vi "IQ Impairments.vi"(0 "data in":T1[](array[typedef])=[{"I"=0.0, "Q"=0.0, "overflow"=FALSE}, {"I"=0.0, "Q"=0.0, "overflow"=FALSE}], 9 "input valid":bool, 11 "acq in":refnum<class "niUSRP Rx DSP v2 FPGA.lvclass">, 12 "ready for output (T)":bool=TRUE) -> (4 "data out":T1[](array[typedef]), 10 "output valid":bool, 14 "ready for input":bool, 15 "acq out":refnum<class "niUSRP Rx DSP v2 FPGA.lvclass">)   [LabVIEW 2025, in "niUSRP Rx DSP v2 FPGA.lvclass"]
uses:
  niUSRP Rx DSP v2 FPGA.lvclass
  <instrlib>/_niInstr/DSP/v1/Shared/Public/IQ Data.ctl
  <instrlib>/_niInstr/DSP Control/Interface/v1/FPGA/IQ Impairments/IQ 18-bit/IQ Impairments Interface (18-bit).lvclass
  <instrlib>/_niInstr/Basic Elements/v1/FPGA/niInstr Basic Elements v1 FPGA.lvlib
  <instrlib>/_niInstr/DSP/v1/Shared/niInstr DSP v1 Shared.lvlib
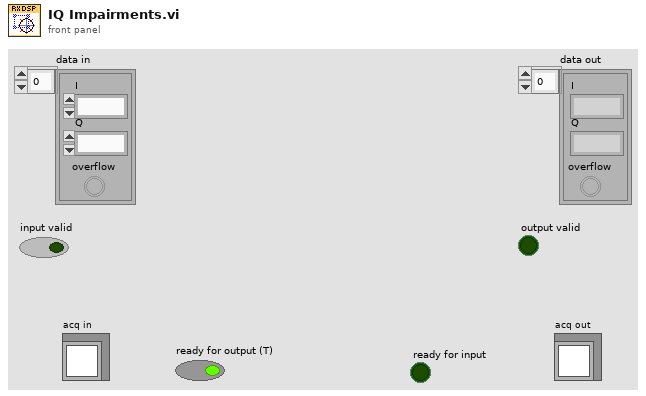
[diagram p1: front panel]
types:
  T1 = typedef "niInstr DSP v1 Shared.lvlib/IQ Data.ctl" = cluster{"I":fxp<+/-,18,1>, "Q":fxp<+/-,18,1>, "overflow":bool}
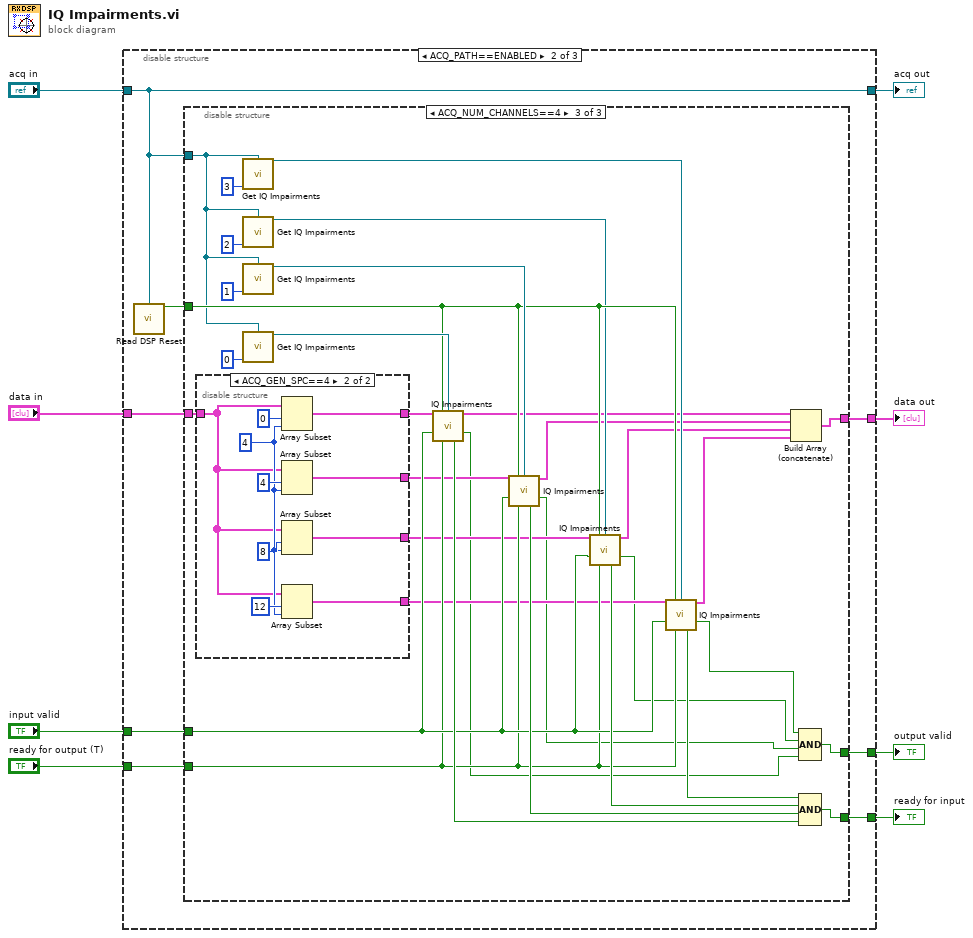
[diagram p0: block diagram]
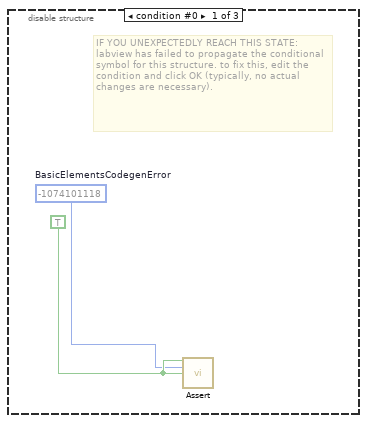
[diagram p2: hidden frame]
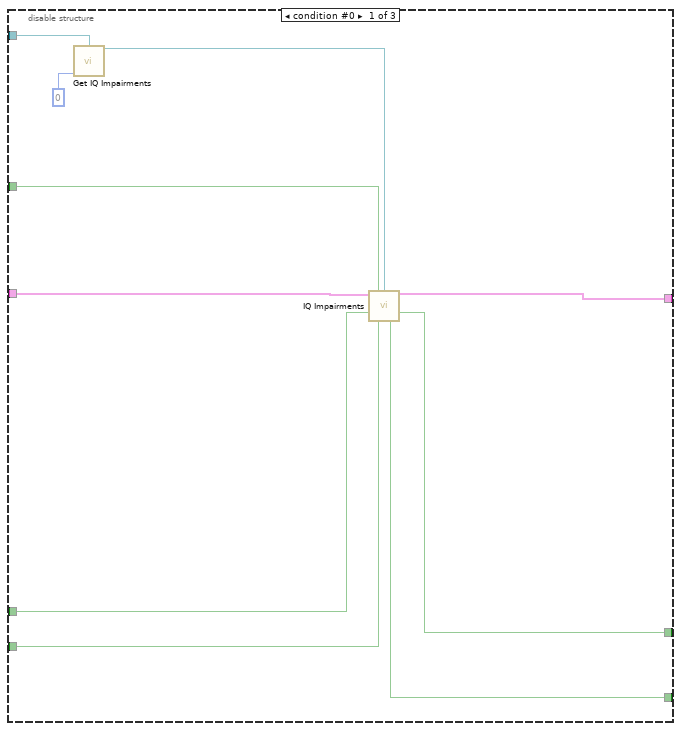
[diagram p3: hidden frame]
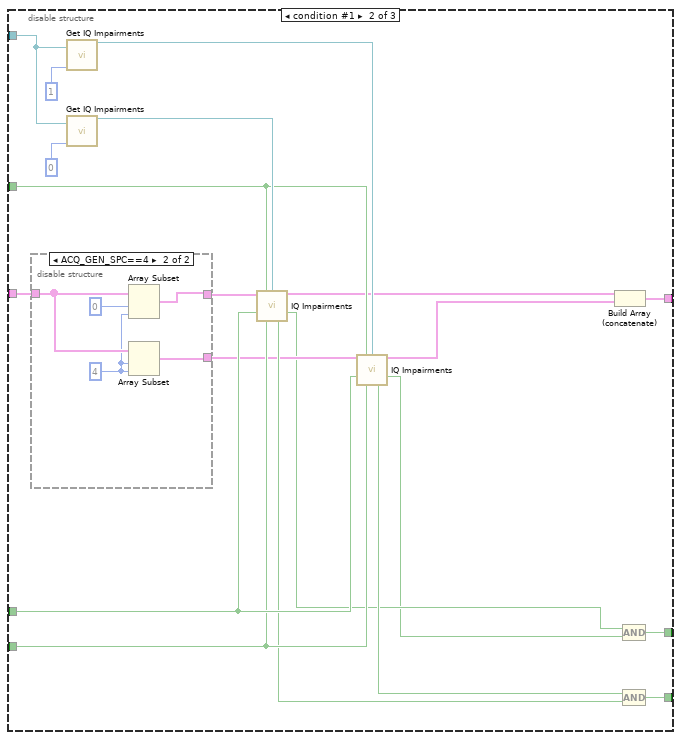
[diagram p4: hidden frame]
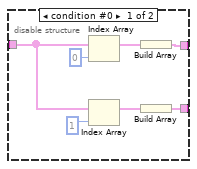
[diagram p5: hidden frame]
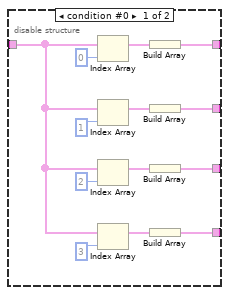
[diagram p6: hidden frame]
diagram:
  n1 = disable-structure shown="ACQ_PATH==ENABLED" {
    disable-tunnel: [_ w18 w118] -> w8
    disable-tunnel: "input valid" -> [_ w17 w116]
    disable-tunnel: "ready for output (T)" -> [_ w16 w117]
    disable-tunnel: [_ w15 w116] -> w5
    disable-tunnel: "acq in" -> [_ w12 w119]
    disable-tunnel: [_ w12 w119] -> w4
    disable-tunnel: "data in" -> [_ w11 w118]
    disable-tunnel: [_ w14 w117] -> w2
    frame condition #0 {
      w10 = TRUE ("assert")
      w9 = -1074101118  # BasicElementsCodegenError
      # "IF YOU UNEXPECTEDLY REACH THIS STATE:\nlabview has failed to propagate the conditional symbol for this structure. to fix this, edit the condition and click OK (typically, no actual changes are necessary)."
      n2 = call <instrlib>:"Assert.vi"("assert"=w10, "error code"=w9, "enable show error"=w10) -> ()  [unwired: 13 in]
    }
    frame condition #1 (active) {
      n3 = call-dynamic "Read DSP Reset.vi"("acq"=w12) -> ("dsp reset"=w13:bool)  [unwired: 14 in]
      n4 = disable-structure shown="ACQ_NUM_CHANNELS==4" {
        disable-tunnel: [w28 w40 w88] -> w18
        disable-tunnel: w17 -> [w27 w42 w76]
        disable-tunnel: w16 -> [w26 w41 w75]
        disable-tunnel: [w25 w39 w87] -> w15
        disable-tunnel: [w24 w38 w86] -> w14
        disable-tunnel: w13 -> [w23 w43 w81]
        disable-tunnel: w12 -> [w21 w45 w74]
        disable-tunnel: w11 -> [w19 w35 w73]
        frame condition #0 {
          n5 = call-dynamic "Get IQ Impairments.vi"("acq in"=w21, "ch"=u8 0) -> ("iq impairments"=w22:refnum<class "IQ Impairments Interface (18-bit).lvclass">)  [unwired: 13 in]
          n6 = call-dynamic "IQ Impairments.vi"("data in"=w19, "reset"=w23, "iq impairments"=w22, "input valid"=w27, "ready for output (T)"=w26) -> ("data out"=w28:T1[], "output valid"=w25:bool, "ready for input"=w24:bool)  [unwired: 7 in, 1 out]
        }
        frame condition #1 {
          n7 = disable-structure shown="ACQ_GEN_SPC==4" {
            disable-tunnel: w35 -> [w51 w58]
            disable-tunnel: [w50 w59] -> w34
            disable-tunnel: [w49 w57] -> w33
            frame condition #0 {
              n8 = Index Array(array=w51, index=0) -> (element=w55:T1)
              n9 = Index Array(array=w51, index=1) -> (element=w53:T1)
              n10 = Build Array(w55) -> (w50:T1[])
              n11 = Build Array(w53) -> (w49:T1[])
            }
            frame condition #1 (active) {
              w56 = 4 ("length")
              n12 = Array Subset(array=w58, index=0, length=w56) -> (w59:T1[])
              n13 = Array Subset(array=w58, index=w56, length=w56) -> (w57:T1[])
            }
          }
          n14 = call-dynamic "Get IQ Impairments.vi"("acq in"=w45, "ch"=u8 1) -> ("iq impairments"=w44:refnum<class "IQ Impairments Interface (18-bit).lvclass">)  [unwired: 13 in]
          n15 = call-dynamic "Get IQ Impairments.vi"("acq in"=w45, "ch"=u8 0) -> ("iq impairments"=w48:refnum<class "IQ Impairments Interface (18-bit).lvclass">)  [unwired: 13 in]
          n16 = call-dynamic "IQ Impairments.vi"("data in"=w34, "reset"=w43, "iq impairments"=w48, "input valid"=w42, "ready for output (T)"=w41) -> ("data out"=w32:T1[], "output valid"=w30:bool, "ready for input"=w37:bool)  [unwired: 7 in, 1 out]
          n17 = call-dynamic "IQ Impairments.vi"("data in"=w33, "reset"=w43, "iq impairments"=w44, "input valid"=w42, "ready for output (T)"=w41) -> ("data out"=w31:T1[], "output valid"=w29:bool, "ready for input"=w36:bool)  [unwired: 7 in, 1 out]
          n18 = Build Array (concatenate)(w32, w31) -> (w40:T1[])
          n19 = Compound Arithmetic op=AND(w30, w29) -> (w39:bool)
          n20 = Compound Arithmetic op=AND(w36, w37) -> (w38:bool)
        }
        frame condition #2 (active) {
          n21 = disable-structure shown="ACQ_GEN_SPC==4" {
            disable-tunnel: [w101 w109] -> w72
            disable-tunnel: [w100 w108] -> w71
            disable-tunnel: [w99 w107] -> w70
            disable-tunnel: w73 -> [w94 w110]
            disable-tunnel: [w93 w106] -> w69
            frame condition #0 {
              n22 = Index Array(array=w94, index=0) -> (element=w105:T1)
              n23 = Index Array(array=w94, index=1) -> (element=w103:T1)
              n24 = Index Array(array=w94, index=2) -> (element=w95:T1)
              n25 = Index Array(array=w94, index=3) -> (element=w97:T1)
              n26 = Build Array(w105) -> (w101:T1[])
              n27 = Build Array(w103) -> (w100:T1[])
              n28 = Build Array(w95) -> (w99:T1[])
              n29 = Build Array(w97) -> (w93:T1[])
            }
            frame condition #1 (active) {
              w111 = 4 ("length")
              n30 = Array Subset(array=w110, index=0, length=w111) -> (w109:T1[])
              n31 = Array Subset(array=w110, index=4, length=w111) -> (w108:T1[])
              n32 = Array Subset(array=w110, index=8, length=w111) -> (w107:T1[])
              n33 = Array Subset(array=w110, index=12, length=w111) -> (w106:T1[])
            }
          }
          n34 = call-dynamic "Get IQ Impairments.vi"("acq in"=w74, "ch"=u8 3) -> ("iq impairments"=w80:refnum<class "IQ Impairments Interface (18-bit).lvclass">)  [unwired: 13 in]
          n35 = call-dynamic "Get IQ Impairments.vi"("acq in"=w74, "ch"=u8 2) -> ("iq impairments"=w79:refnum<class "IQ Impairments Interface (18-bit).lvclass">)  [unwired: 13 in]
          n36 = call-dynamic "Get IQ Impairments.vi"("acq in"=w74, "ch"=u8 1) -> ("iq impairments"=w89:refnum<class "IQ Impairments Interface (18-bit).lvclass">)  [unwired: 13 in]
          n37 = call-dynamic "Get IQ Impairments.vi"("acq in"=w74, "ch"=u8 0) -> ("iq impairments"=w92:refnum<class "IQ Impairments Interface (18-bit).lvclass">)  [unwired: 13 in]
          n38 = call-dynamic "IQ Impairments.vi"("data in"=w72, "reset"=w81, "iq impairments"=w92, "input valid"=w76, "ready for output (T)"=w75) -> ("data out"=w68:T1[], "output valid"=w61:bool, "ready for input"=w85:bool)  [unwired: 7 in, 1 out]
          n39 = call-dynamic "IQ Impairments.vi"("data in"=w71, "reset"=w81, "iq impairments"=w89, "input valid"=w76, "ready for output (T)"=w75) -> ("data out"=w67:T1[], "output valid"=w62:bool, "ready for input"=w84:bool)  [unwired: 7 in, 1 out]
          n40 = call-dynamic "IQ Impairments.vi"("data in"=w70, "reset"=w81, "iq impairments"=w79, "input valid"=w76, "ready for output (T)"=w75) -> ("data out"=w66:T1[], "output valid"=w63:bool, "ready for input"=w77:bool)  [unwired: 7 in, 1 out]
          n41 = call-dynamic "IQ Impairments.vi"("data in"=w69, "reset"=w81, "iq impairments"=w80, "input valid"=w76, "ready for output (T)"=w75) -> ("data out"=w65:T1[], "output valid"=w64:bool, "ready for input"=w78:bool)  [unwired: 7 in, 1 out]
          n42 = Build Array (concatenate)(w68, w67, w66, w65) -> (w88:T1[])
          n43 = Compound Arithmetic op=AND(w64, w63, w62, w61) -> (w87:bool)
          n44 = Compound Arithmetic op=AND(w78, w77, w84, w85) -> (w86:bool)
        }
      }
    }
    frame condition #2 {
    }
  }
  "data out" <- w8
  "output valid" <- w5
  "ready for input" <- w2
  "acq out" <- w4
